vi "DAQ C(T) Analog In Manager.vi"(0 "channel (single point) (0)":tag="Dev1/ai0", 1 "AI mode chooser":T1(ring), 5 "Channels (Triggered Waveform)":tag[](array[tag])=["Dev1/ai1", "Dev1/ai2"], 9 "number of scans to acquire":i32=1000, 11 "error in (no error)":errorcluster, 12 "scan rate":dbl=100000.0 format="%.2f", 13 "trigger edge":i32(ring)=10171 items=["Rising"=10280, "Falling"=10171], 14 "trigger level":dbl=2.5 format="%.2f") -> (3 "Timed Out":bool, 6 "V meas":dbl=0.0048828125 format="%.2f", 8 "data":waveform(dbl)[](array[waveform])=[{"t0"=timestamp(3087584082.493 s since 1904-01-01), "dt"=1.9999999494757503e-05, "Y"=[]}, {"t0"=timestamp(3087584082.493 s since 1904-01-01), "dt"=1.9999999494757503e-05, "Y"=array[1000 elements]}], 15 "error out":errorcluster)   [LabVIEW 2013]
doc: "this vi allows for either single point acq from a single channel \nor buffered & triggered waveform acq from multiple channels\n\nMatt Strader\nPaul K Dixon\nPhysics 350\nCSUSB Physics"
panel:
  # "General Controls"
  # "DAQ C(T) Analog In Acquisition Manager"
  # "Single Point Mode"
  # "Triggered Waveform Mode"
  # "Error I/O"
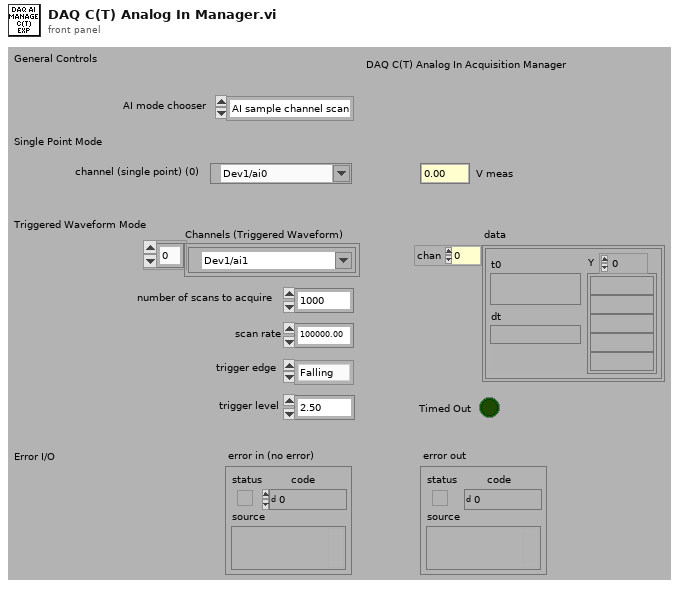
[diagram p1: front panel]
types:
  T1 = enum16{"AI sample channel scan", "AI Waveform triggered"}
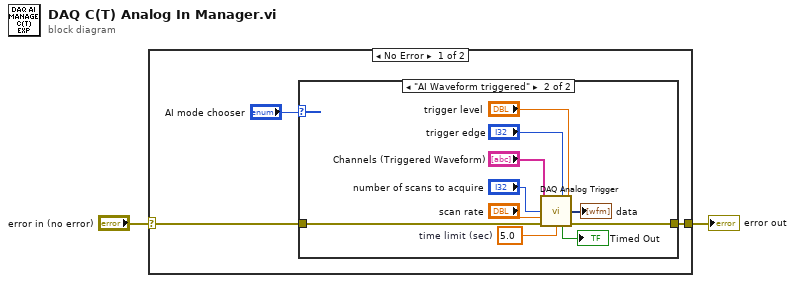
[diagram p0: block diagram]
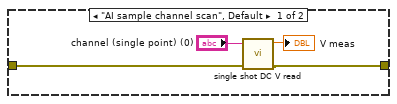
[diagram p2: hidden frame]
diagram:
  n1 = case shown="No Error" "error in (no error)" {
    selector: "error in (no error)" -> [w3 w20]
    tunnel: [w4 w20] -> w1
    frame No Error {
      n2 = case shown="\"AI Waveform triggered\"" "AI mode chooser" {
        tunnel: w3 -> [w8 w19]
        tunnel: [w9 w18] -> w4
        frame "AI sample channel scan", Default {
          n3 = call "single shot DC V read.vi"("error in"=w8, "DAQmx Physical Channel"="channel (single point) (0)") -> ("error out"=w9:errorcluster, "data"=→"V meas":dbl)  [unwired: 1 in, 5 out]
        }
        frame "AI Waveform triggered" {
          w15 = 5.0  # time limit (sec)
          n4 = call "DAQ Analog Trigger.vi"("Channels"="Channels (Triggered Waveform)", "trigger edge"="trigger edge", "trigger level"="trigger level", "number of samples"="number of scans to acquire", "rate"="scan rate", "error in"=w19, "timeout (s)"=w15) -> ("data"=→"data":dynamicdata, "Timed Out"=→"Timed Out":bool, "error out"=w18:errorcluster)  [unwired: 3 in, 3 out]
        }
      }
    }
    frame Error {
    }
  }
  "error out" <- w1
